vi "Enable Custom Device.vi"(8 "error in (no error)":errorcluster, 11 "AIM ARINC 429 ref":T1 format="%.0x") -> (0 "error out":errorcluster, 3 "AIM ARINC 429 ref out":T1 format="%.0x")   [LabVIEW 2020, in "AIM ARINC 429 Scripting.lvlib"]
doc: "Enables an AIM ARINC 429 custom device."
uses:
  AIM ARINC 429 Scripting.lvlib
  <vilib>/NI VeriStand/Custom Device API/Custom Device API.lvlib
  NationalInstruments.VeriStand.SystemDefinitionAPI
  Constants.vi
  <vilib>/NI VeriStand/Custom Device API/Custom Device Item Ref.ctl
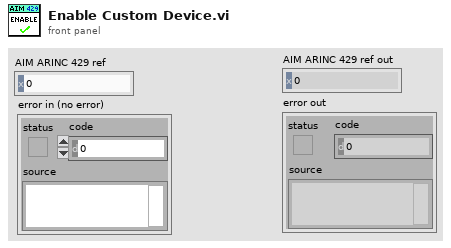
[diagram p1: front panel]
types:
  T1 = typedef "Custom Device API.lvlib/Custom Device Item Ref.ctl" = u64
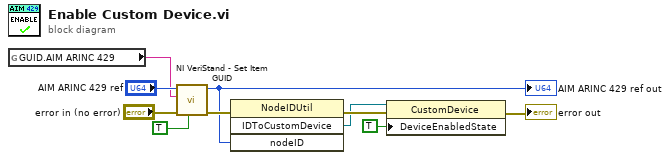
[diagram p0: block diagram]
diagram:
  n1 = global read "Constants.vi" "GUID.AIM ARINC 429"() -> (w1:string)
  n2 = call <vilib>:"NI VeriStand - Set Item GUID.vi"("Refresh System Explorer Tree? (F)"=TRUE, "error in (no error)"="error in (no error)", "GUID"=w1, "Item Ref in"="AIM ARINC 429 ref") -> ("error out"=w10:errorcluster, "Item Ref out"=w4:T1)  [unwired: 6 in]
  "AIM ARINC 429 ref out" <- w4
  n3 = invoke class="NodeIDUtil" method="IDToCustomDevice"(error in=w10, "nodeID"=w4) -> (error out=w9:errorcluster, "IDToCustomDevice"=w7:refnum<k24>)  [unwired: 2 in, 2 out]
  n4 = property class="CustomDevice"(reference=w7, error in=w9, "DeviceEnabledState"=TRUE) -> (error out=→"error out":errorcluster)  [unwired: 1 out]
